vi "Joystick to Velocity Control.vi"(8 "Error In":errorcluster, 11 "Aircraft ID":u8) -> (0 "Error Out":errorcluster, 2 "Velocity Message":u8[](array[numeric]), 3 "output cluster":T1)   [LabVIEW 2014]
uses:
  Aircraft Information/Sub VI/Get Aircraft RC.vi
  Joystick/FGVs/Joystick Input/Method VIs/Get Joystick Input.vi
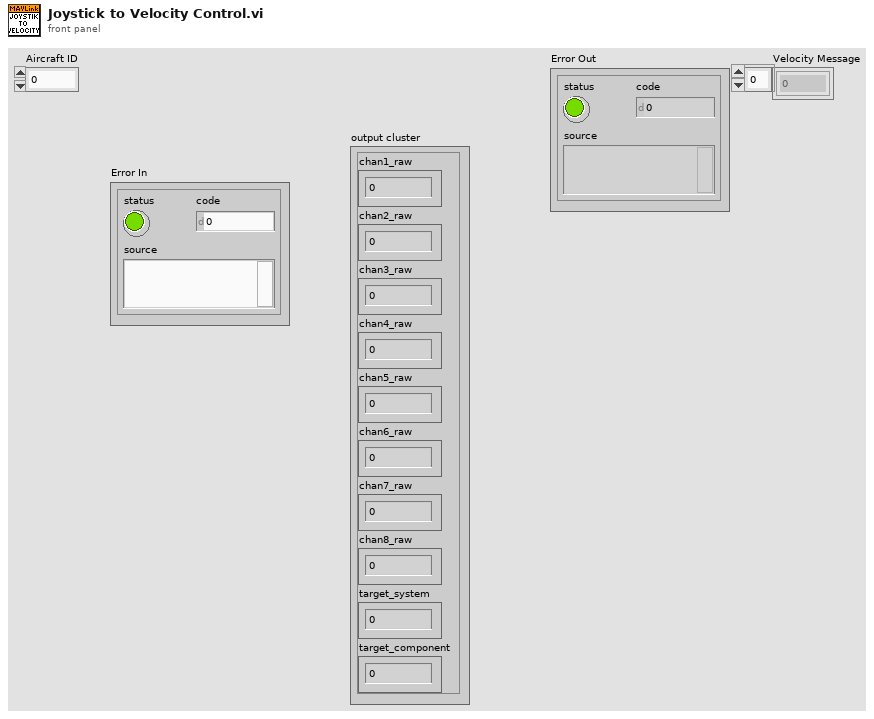
[diagram p1: front panel]
types:
  T1 = cluster{"chan1_raw":u16, "chan2_raw":u16, "chan3_raw":u16, "chan4_raw":u16, "chan5_raw":u16, "chan6_raw":u16, "chan7_raw":u16, "chan8_raw":u16, "target_system":u8, "target_component":u8}
  T2 = typedef "Joystick Input.ctl" = cluster{"Roll (%)":dbl, "Pitch (%)":dbl, "Yaw (%)":dbl, "Throttle (%)":dbl, "Brake":bool, "Emergency Stop":bool, "Arm":bool, "Disarm":bool}
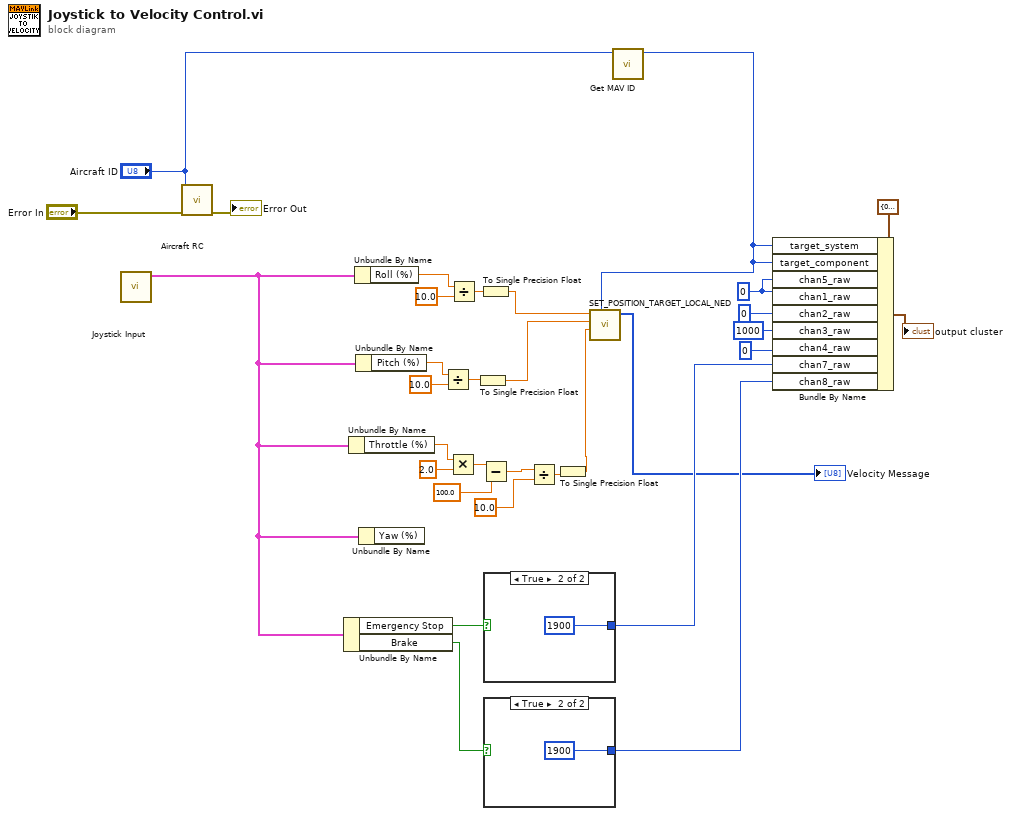
[diagram p0: block diagram]
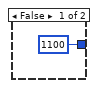
[diagram p2: hidden frame]
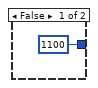
[diagram p3: hidden frame]
diagram:
  w1 = u16 0 ("chan1_raw")
  n1 = call-poly "Joystick Input.vi"() -> ("Joystick Input Out"=w24:T2)  [unwired: 11 in]
  n2 = call-poly "Aircraft RC.vi"("Error In"="Error In", "Aircraft ID"="Aircraft ID") -> ("Error Out"=→"Error Out":errorcluster)  [unwired: 8 in, 1 out]
  n3 = Unbundle By Name(w24) -> ("Emergency Stop"=w31:bool, "Brake"=w27:bool)
  n4 = Unbundle By Name(w24) -> ("Throttle (%)"=w13:dbl)
  n5 = Unbundle By Name(w24) -> ("Roll (%)"=w18:dbl)
  n6 = Unbundle By Name(w24) -> ("Pitch (%)"=w15:dbl)
  n7 = Unbundle By Name(w24) -> ()  [unwired: 1 out]
  n8 = Divide(x=w15, y=10.0) -> (x/y=w11:dbl)
  n9 = Multiply(x=w13, y=2.0) -> (x*y=w7:dbl)
  n10 = Divide(x=w18, y=10.0) -> (x/y=w12:dbl)
  n11 = To Single Precision Float(number=w11) -> (single precision float=w9:sgl)
  n12 = To Single Precision Float(number=w12) -> (single precision float=w10:sgl)
  n13 = Subtract(x=w7, y=100.0) -> (x-y=w5:dbl)
  n14 = case shown="True" w31 {
    tunnel: [u16 1100 u16 1900] -> w28
    frame False {
    }
    frame True {
    }
  }
  n15 = case shown="True" w27 {
    tunnel: [u16 1100 u16 1900] -> w26
    frame False {
    }
    frame True {
    }
  }
  n16 = Divide(x=w5, y=10.0) -> (x/y=w3:dbl)
  n17 = To Single Precision Float(number=w3) -> (single precision float=w2:sgl)
  n18 = call "Get MAV ID.vi"("Aircraft Index"="Aircraft ID") -> ("Aircraft ID"=w19:u8)  [unwired: 10 in]
  n19 = call "SET_POSITION_TARGET_LOCAL_NED.vi"("MAV ID"=w19, "vz"=w2, "vy"=w9, "vx"=w10) -> ("MAVLink Message"=→"Velocity Message":u8[])  [unwired: 7 in]
  n20 = Bundle By Name(cluster=T1 {"chan1_raw"=0, "chan2_raw"=0, "chan3_raw"=0, "chan4_raw"=0, "chan5_raw"=0, "chan6_raw"=0, "chan7_raw"=0, "chan8_raw"=0, "target_system"=0, "target_component"=0} ("Payload"), "target_system"=w19, "target_component"=w19, "chan5_raw"=w1, "chan1_raw"=w1, "chan2_raw"=u16 0, "chan3_raw"=u16 1000, "chan4_raw"=u16 0, "chan7_raw"=w28, "chan8_raw"=w26) -> (→"output cluster":T1)
